vi "Variant to Formatted String.vi"(6 "Indentation String (4-space)":string, 8 "Error In":errorcluster, 9 "Hide Long Cluster Names (T)":bool=TRUE, 10 "Variant":variant, 11 "Label":string) -> (0 "Error Out":errorcluster, 3 "String":string)   [LabVIEW 2021, in "Variant.lvlib"]
uses:
  Variant.lvlib
  <vilib>/Utility/config.llb/NI_LVConfig.lvlib
  <userlib>/_OpenG.lib/file/file.llb/openg_file.lvlib
  <userlib>/_OpenG.lib/variantconfig/variantconfig.llb/openg_variant_configuration_file.lvlib
  Strings/Strings.lvlib
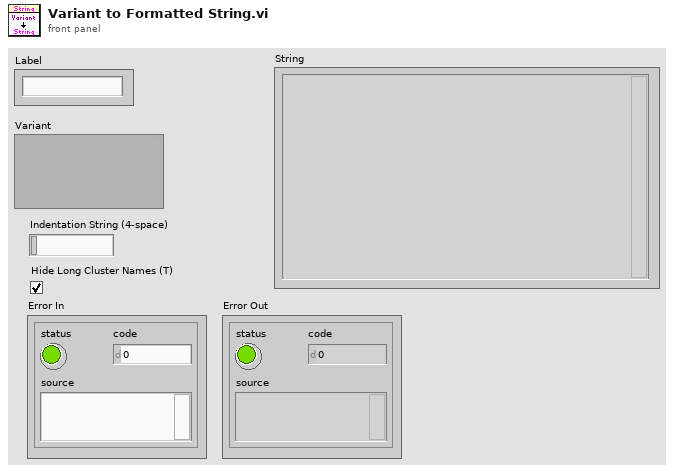
[diagram p1: front panel]
types:
  T1 = typedef "NI_LVConfig.lvlib/Config Data RefNum.ctl" = refnum<k1>
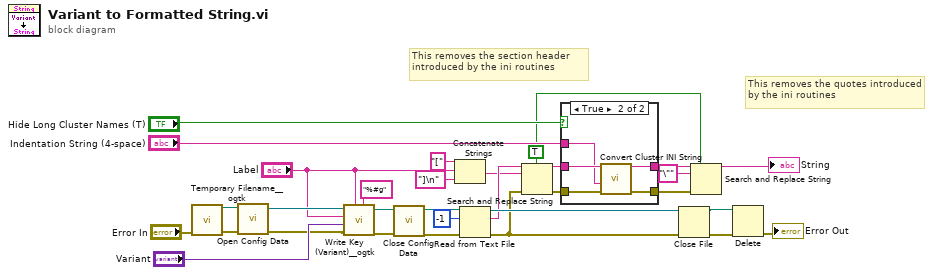
[diagram p0: block diagram]
diagram:
  w1 = TRUE ("replace all? (F)")
  # "This removes the quotes introduced by the ini routines"
  # "This removes the section header introduced by the ini routines"
  n1 = call <userlib>:"Temporary Filename__ogtk.vi"("error in (no error)"="Error In") -> ("error out"=w19:errorcluster, "file in tmp dir"=w18:path)  [unwired: 5 in]
  n2 = call <vilib>:"Open Config Data.vi"("error in (no error)"=w19, "configuration file path"=w18) -> ("error out"=w20:errorcluster, "refnum"=w22:T1)  [unwired: 7 in, 1 out]
  n3 = call <userlib>:"Write Key (Variant)__ogtk.vi"("float number format"="%#g", "section"="Label", "error in (no error)"=w20, "key-value"="Variant", "key (optional)"="Label", "refnum"=w22) -> ("error out"=w24:errorcluster, "refnum out"=w25:T1)  [unwired: 4 in]
  n4 = call <vilib>:"Close Config Data.vi"("error in (no error)"=w24, "refnum"=w25) -> ("error out"=w27:errorcluster, "file path"=w26:path)  [unwired: 8 in]
  n5 = Concatenate Strings("[" ("string"), "Label", "]\n" ("string")) -> (w12:string)
  n6 = Read from Text File(file (use dialog)=w26, count=-1, error in=w27) -> (refnum out=w29:refnum<file>, text=w13:string, error out=w3:errorcluster)  [unwired: 1 in, 1 out]
  n7 = Search and Replace String(replace all?=w1, input string=w13, search string=w12, error in=w3) -> (result string=w8:string, error out=w5:errorcluster)  [unwired: 4 in, 2 out]
  n8 = case shown="True" "Hide Long Cluster Names (T)" {
    tunnel: w8 -> [w33 w38]
    tunnel: [w33 w37] -> w7
    tunnel: w5 -> [w32 w36]
    tunnel: [w32 w35] -> w4
    tunnel: "Indentation String (4-space)" -> [_ w34]
    frame False {
    }
    frame True {
      n9 = call "Convert Cluster INI String.vi"("error in (no error)"=w36, "Indentation String (4-space)"=w34, "string in"=w38) -> ("error out"=w35:errorcluster, "string out"=w37:string)  [unwired: 7 in]
    }
  }
  n10 = Close File(refnum=w29, error in=w3) -> (path=w31:path, error out=w30:errorcluster)
  n11 = Search and Replace String(replace all?=w1, input string=w7, search string="\"", error in=w4) -> (result string=→"String":string)  [unwired: 4 in, 3 out]
  n12 = Delete(path (use dialog)=w31, error in=w30) -> (error out=→"Error Out":errorcluster)  [unwired: 3 in, 2 out]
